vi "testCANopen.vi"() -> ()   [LabVIEW 2017, in "canopen.lvlib"]
doc: "Tests CANopen (and possibly CANbus) nets exercising the CANopen.lvclass APIs."
uses:
  canopen.lvlib
  CANopen/Multiplexor.ctl
  CANopen/FunctionCode.ctl
  DSP402/DSP402.lvclass
  CANopen/CANopen.lvclass
  DSP402/DriveState.ctl
  DSP402/DriveMode.ctl
  types/threestateFlag.ctl
panel:
  in  "CANopen":refnum<class "CANopen.lvclass">
  in  "DSP402":refnum<class "DSP402.lvclass">
  in  "Variant":variant=variant(u8[] [80, 0])
  in  "Tab Control":T1(tab)
  in  "NMT send":bool
  in  "Node ID (NMT)":u8=50 caption="Node ID"
  in  "Command specifier":u8(ring)=129 items=["Start remote node"=1, "Stop remote node"=2, "Enter pre-operational state"=128, "Reset node"=129, "Reset communication"=130]
  in  "SDO size":u8=2 caption="Bytes" format="%0d"
  in  "SDO read":bool
  in  "Multiplexor":T2={"Index"=4119, "Sub-index"=0} {"Sub-index" format="%02x"; "Index" format="%04x"}
  in  "SDO value":u32 caption="Value" format="%08x"
  in  "SDO write":bool
  in  "Node ID (SDO)":u8=50 caption="Node ID"
  in  "Remap TxPDO":bool
  in  "TxPDO map":cluster{"CobID":u32, "nBytes":u8}[](array[cluster])=[{"CobID"=434, "nBytes"=2}] {"CobID" format="%x"}
  out "Input image":bool[](array[boolean])
  in  "Remap RxPDO":bool
  in  "RxPDO map":cluster{"CobID":u32, "nBytes":u8}[](array[cluster])=[{"CobID"=562, "nBytes"=5}] {"CobID" format="%x"}
  in  "Output image":bool[](array[boolean])
  in  "Node ID (402)":u8 caption="Node ID"
  in  "State (402)":T3 caption="State"
  in  "Mode (402)":T4 caption="Mode" items=["Undefined"=0, "Profile Position Mode"=1, "Velocity Mode"=2, "Profile Velocity Mode"=3, "Torque Profile Mode"=4, "Homing Mode"=6, "Interpolated Position Mode"=7]
  in  "Position (402)":u32 caption="Position"
  in  "Speed (402)":i16=500 caption="Speed (RpM)"
  in  "Operation flags (402)":cluster{"ON":bool, "OFF":bool}[](array[cluster])=[{"ON"=FALSE, "OFF"=FALSE}, {"ON"=FALSE, "OFF"=FALSE}, {"ON"=FALSE, "OFF"=FALSE}, {"ON"=FALSE, "OFF"=FALSE}] caption="Force bit 4, 5, 6 and Halt"
  in  "Acceleration (402)":u32=100 caption="Acc"
  in  "Deceleration (402)":u32=100 caption="Dec"
  in  "Get status (402)":bool
  in  "PDO unlink":bool
  in  "PDO link":bool
  in  "Node ID (link)":u8=50 caption="Node ID"
  in  "Function code (link)":T5=4 caption="Function code" items=["NMT", "SYNC", "TIME STAMP", "EMERGENCY", "PDO1 (tx)", "PDO1 (rx)", "PDO2 (tx)", "PDO2 (rx)", "PDO3 (tx)", "PDO3 (rx)", "PDO4 (tx)", "PDO4 (rx)", "SDO (tx)", "SDO (rx)", "NMT Error Control"]
  in  "Indices":cluster{"Communication":u32, "Mapping":u32}={"Communication"=6144, "Mapping"=6656} {"Mapping" format="%x"; "Communication" format="%x"}
  in  "Map":cluster{"Multiplexor":T2, "nBits":u8}[](array[cluster])=[{"Multiplexor"={"Index"=24832, "Sub-index"=1}, "nBits"=16}] {"Multiplexor"."Sub-index" format="%02x"; "Multiplexor"."Index" format="%04x"}
  in  "Heartbeat set":bool
  in  "Heartbeat table":T6(array[cluster]) {"Period" format="%#.3g"}
  in  "Raw send":bool
  in  "Data (raw)":u8[](array[numeric]) caption="Data" format="%02x"
  in  "Node ID (raw)":u8 caption="Node ID"
  in  "Function code (raw)":T5=1 items=["NMT", "SYNC", "TIME STAMP", "EMERGENCY", "PDO1 (tx)", "PDO1 (rx)", "PDO2 (tx)", "PDO2 (rx)", "PDO3 (tx)", "PDO3 (rx)", "PDO4 (tx)", "PDO4 (rx)", "SDO (tx)", "SDO (rx)", "NMT Error Control"]
  in  "Stop":bool
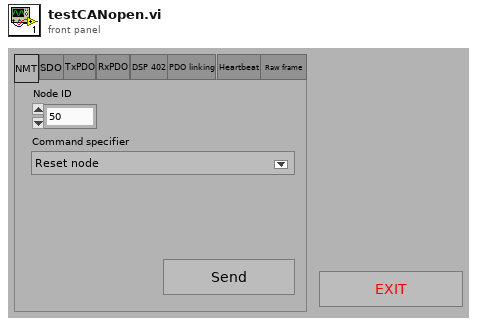
[diagram p1: front panel]
types:
  T1 = enum32{"NMT", "SDO", "TxPDO", "RxPDO", "DSP 402", "PDO linking", "Heartbeat", "Raw frame"}
  T2 = typedef "canopen.lvlib/CANopen.lvclass/Multiplexor.ctl" = cluster{"Index":u16, "Sub-index":u8}
  T3 = typedef "canopen.lvlib/DSP402.lvclass/DriveState.ctl" = enum16{"Start", "Not ready to switch on", "Switch on disabled", "Ready to switch on", "Switched on", "Operation enable", "Fault reaction active", "Fault", "Quick stop active"}
  T4 = typedef "canopen.lvlib/DSP402.lvclass/DriveMode.ctl" = i8
  T5 = typedef "canopen.lvlib/CANopen.lvclass/FunctionCode.ctl" = u8
  T6 = cluster{"Node ID":u8, "Period":dbl, "Set value":i16, "Value":i16}[]
  T7 = typedef "canopen.lvlib/threestateFlag.ctl" = i8
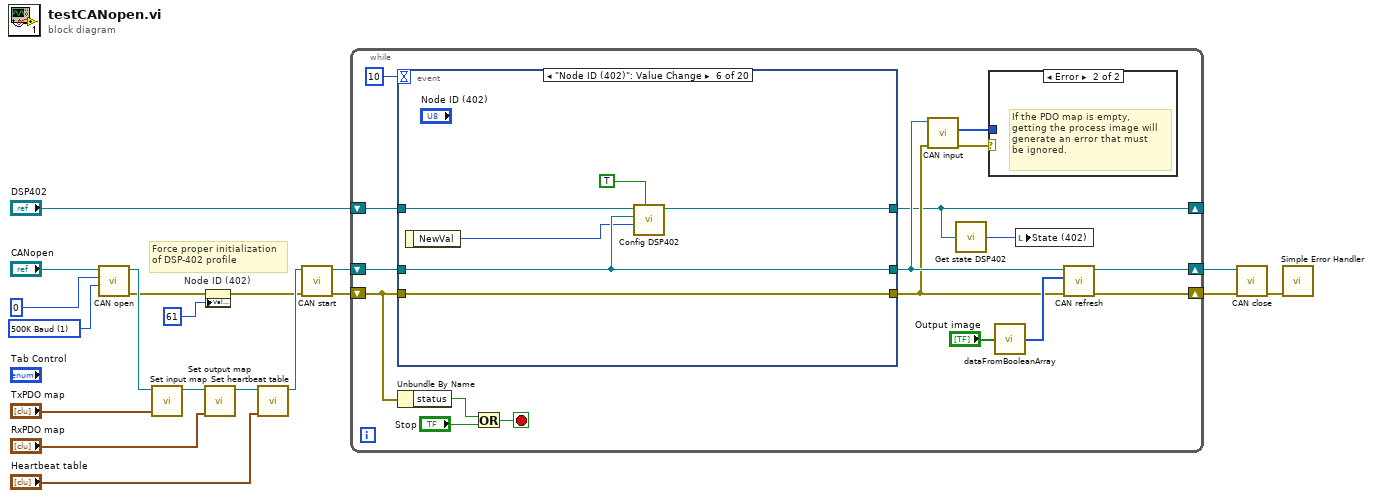
[diagram p0: block diagram]
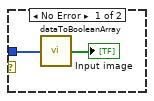
[diagram p2: hidden frame]
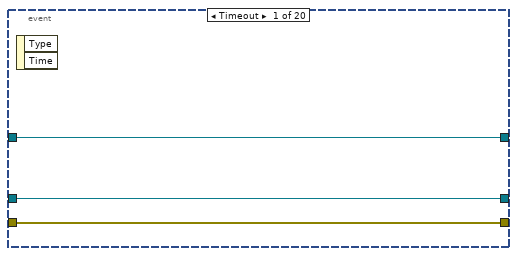
[diagram p3: hidden frame]
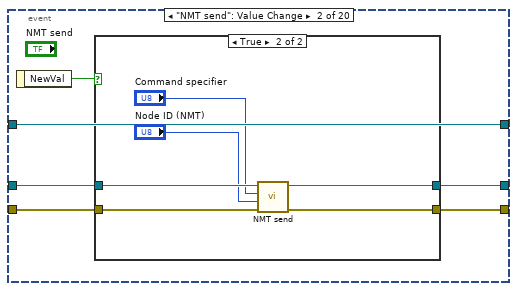
[diagram p4: hidden frame]
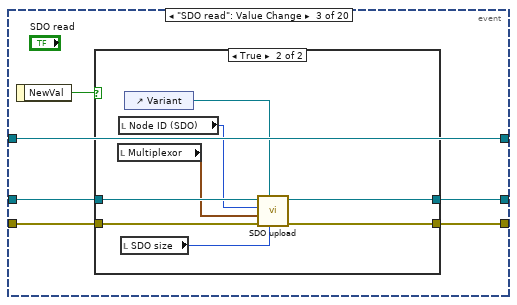
[diagram p6: hidden frame]
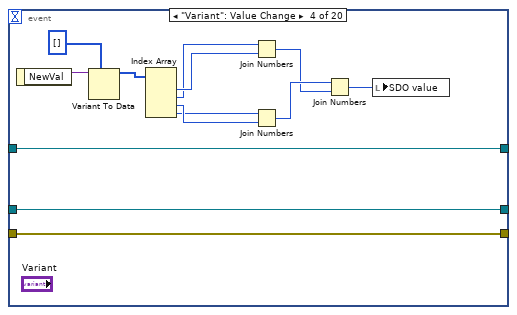
[diagram p8: hidden frame]
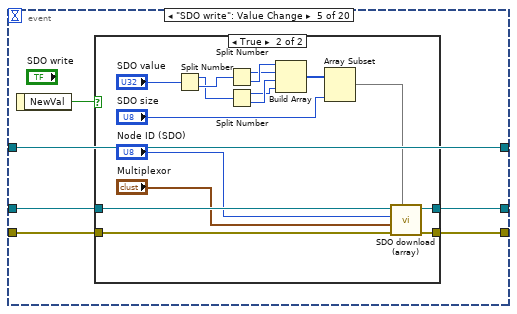
[diagram p9: hidden frame]
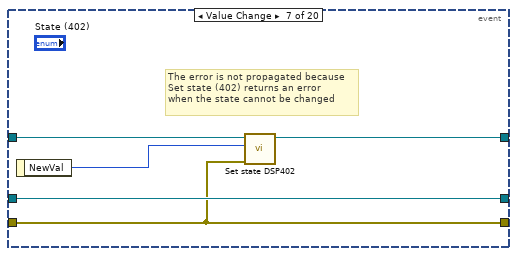
[diagram p11: hidden frame]
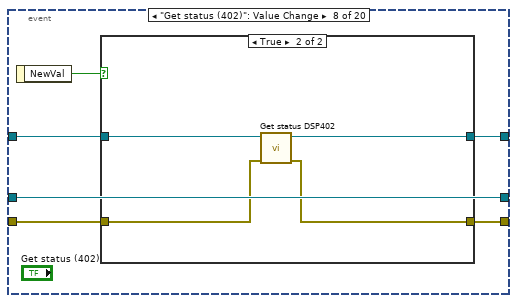
[diagram p12: hidden frame]
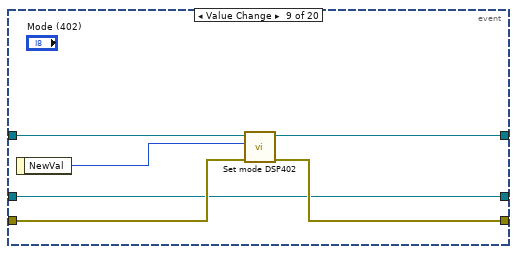
[diagram p14: hidden frame]
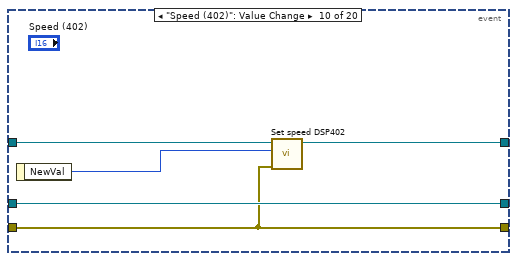
[diagram p15: hidden frame]
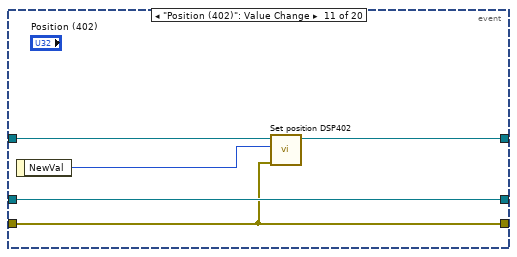
[diagram p16: hidden frame]
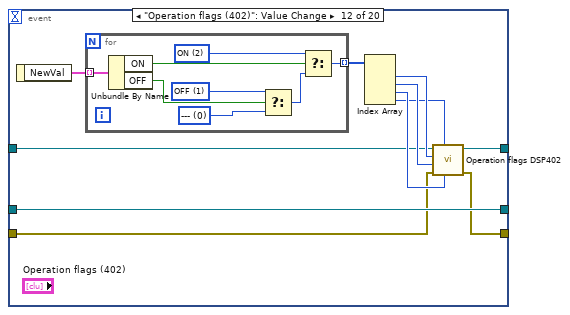
[diagram p17: hidden frame]
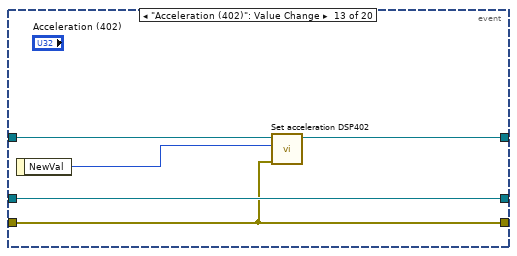
[diagram p18: hidden frame]
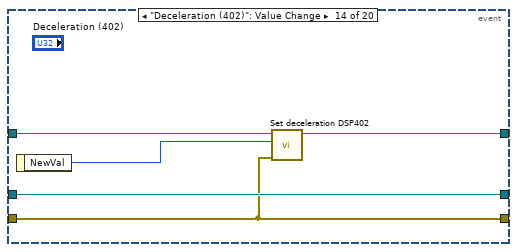
[diagram p19: hidden frame]
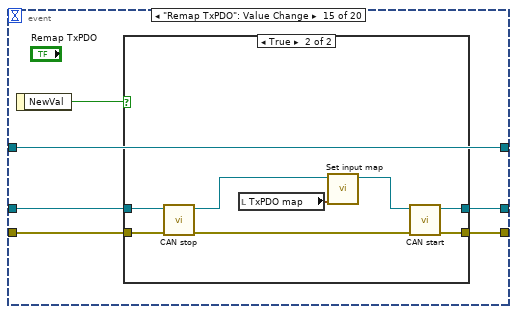
[diagram p20: hidden frame]
diagram:
  w15 = 1 items=["1M Baud", "500K Baud", "250K Baud", "125K Baud", "100K Baud", "62K Baud", "50K Baud"] ("Baud rate")
  # "Force proper initialization\nof DSP-402 profile"
  n1 = call "CAN open.vi"("Baud rate"=w15, "Channel"=u32 0, "CANopen in"="CANopen") -> ("error out"=w3:errorcluster, "CANopen out"=w11:refnum<class "CANopen.lvclass">)  [unwired: 1 in, 2 out]
  n2 = call "Set input map.vi"("Map"="TxPDO map", "CANopen in"=w11) -> ("CANopen out"=w10:refnum<class "CANopen.lvclass">)  [unwired: 5 out]
  n3 = call "Set output map.vi"("Map"="RxPDO map", "CANopen in"=w10) -> ("CANopen out"=w8:refnum<class "CANopen.lvclass">)  [unwired: 5 out]
  n4 = property on="Node ID (402)" class="DigNum (strict)"(error in=w3, "Val(Sgnl)"=u8 61 ("Value (Signaling)")) -> (error out=w2:errorcluster)  [unwired: 1 in, 1 out]
  n5 = call "Set heartbeat table.vi"("Heartbeat table"="Heartbeat table", "CANopen in"=w8) -> ("CANopen out"=w6:refnum<class "CANopen.lvclass">)  [unwired: 1 in, 4 out]
  n6 = call "CAN start.vi"("error in (no error)"=w2, "CANopen in"=w6) -> ("error out"=w5:errorcluster, "CANopen out"=w12:refnum<class "CANopen.lvclass">)  [unwired: 4 out]
  n7 = while {
    shift-right: [w26] -> w18
    shift-left: w5 -> [w34]
    shift-right: [w25] -> w19
    shift-left: w12 -> [w36]
    shift-right: [w21] -> _
    shift-left: "DSP402" -> [w22]
    stop <- w33 stop-if-true
    n8 = event shown="[5] \"Node ID (402)\": Value Change" {
      selector: _ -> [_ _ _ _ _ _ _ _ _ _ _ _ _ _ _ _ _ _ _ _]
      dyn-events: _ -> [_ _ _ _ _ _ _ _ _ _ _ _ _ _ _ _ _ _ _ _]
      timeout: 10 -> [_ _ _ _ _ _ _ _ _ _ _ _ _ _ _ _ _ _ _ _]
      tunnel: [w41 w47 w61 w84 w90 w112 w119 w120 w135 w142 w147 w157 w171 w176 w182 w198 w214 w226 w243 w259] -> w24
      tunnel: w36 -> [w41 w46 w60 w84 w89 w112 w119 w120 w135 w142 w147 w157 w171 w176 w181 w197 w213 w225 w242 w258]
      tunnel: [w40 w45 w59 w83 w88 w110 w115 w125 w136 w138 w143 w150 w167 w172 w180 w196 w212 w224 w241 w257] -> w23
      tunnel: w34 -> [w40 w44 w58 w83 w87 w110 w115 w124 w137 w138 w143 w151 w167 w172 w179 w195 w211 w223 w240 w256]
      tunnel: w22 -> [w39 w42 w56 w72 w85 w114 w117 w121 w133 w140 w146 w148 w169 w174 w177 w193 w209 w221 w238 w254]
      tunnel: [w39 w42 w56 w72 w85 w113 w116 w122 w132 w139 w145 w149 w168 w173 w177 w193 w209 w221 w238 w254] -> w21
      event Timeout {
        n9 = event-data() -> ()  [unwired: 3 out]
      }
      event "NMT send": Value Change {
        n10 = event-data() -> ("NewVal"=w43:bool)  [unwired: 1 out]
        n11 = case shown="True" w43 {
          tunnel: [w49 w52] -> w47
          tunnel: w46 -> [w49 w55]
          tunnel: [w48 w53] -> w45
          tunnel: w44 -> [w48 w54]
          frame False {
          }
          frame True {
            n12 = call "NMT send.vi"("error in (no error)"=w54, "Node ID"="Node ID (NMT)", "Command specifier"="Command specifier", "CANopen in"=w55) -> ("error out"=w53:errorcluster, "CANopen out"=w52:refnum<class "CANopen.lvclass">)  [unwired: 1 in, 1 out]
          }
        }
      }
      event "SDO read": Value Change {
        n13 = event-data() -> ("NewVal"=w57:bool)  [unwired: 1 out]
        n14 = case shown="True" w57 {
          tunnel: [w63 w68] -> w61
          tunnel: w60 -> [w63 w71]
          tunnel: [w62 w69] -> w59
          tunnel: w58 -> [w62 w70]
          frame False {
          }
          frame True {
            n15 = local read "Multiplexor"() -> (w66:T2)
            n16 = local read "Node ID (SDO)"() -> (w67:u8)
            n17 = local read "SDO size"() -> (w64:u8)
            n18 = control-ref of="Variant"() -> (w65:refnum<vi>)
            n19 = call "SDO upload.vi"("Size"=w64, "Destination"=w65, "error in (no error)"=w70, "Multiplexor"=w66, "Node ID"=w67, "CANopen in"=w71) -> ("error out"=w69:errorcluster, "CANopen out"=w68:refnum<class "CANopen.lvclass">)  [unwired: 2 out]
          }
        }
      }
      event "Variant": Value Change {
        n20 = event-data() -> ("NewVal"=w81:variant)  [unwired: 1 out]
        n21 = Variant To Data(type=u8[] [] ("Data"), Variant=w81) -> (data=w79:u8[])  [unwired: 1 in, 1 out]
        n22 = Index Array(array=w79) -> (element #1=w78:u8, element #2=w77:u8, element #3=w76:u8, element #4=w75:u8)  [unwired: 4 in]
        n23 = Join Numbers(hi=w77, lo=w78) -> ((hi.lo)=w73:u16)
        n24 = Join Numbers(hi=w75, lo=w76) -> ((hi.lo)=w74:u16)
        n25 = Join Numbers(hi=w74, lo=w73) -> ((hi.lo)=w80:u32)
        n26 = local write "SDO value"(w80) -> ()
      }
      event "SDO write": Value Change {
        n27 = event-data() -> ("NewVal"=w86:bool)  [unwired: 1 out]
        n28 = case shown="True" w86 {
          tunnel: [w92 w105] -> w90
          tunnel: w89 -> [w92 w108]
          tunnel: [w91 w106] -> w88
          tunnel: w87 -> [w91 w107]
          frame False {
          }
          frame True {
            n29 = Split Number(x="SDO value") -> (hi(x)=w99:u16, lo(x)=w101:u16)
            n30 = Split Number(x=w101) -> (hi(x)=w98:u8, lo(x)=w100:u8)
            n31 = Split Number(x=w99) -> (hi(x)=w96:u8, lo(x)=w97:u8)
            n32 = Build Array(w100, w98, w97, w96) -> (w95:u8[])
            n33 = Array Subset(array=w95, length="SDO size") -> (w93:u8[])  [unwired: 1 in]
            n34 = call "SDO download (array).vi"("Value"=w93, "error in (no error)"=w107, "Multiplexor"="Multiplexor", "Node ID"="Node ID (SDO)", "CANopen in"=w108) -> ("error out"=w106:errorcluster, "CANopen out"=w105:refnum<class "CANopen.lvclass">)  [unwired: 1 in, 2 out]
          }
        }
      }
      event "Node ID (402)": Value Change {
        n35 = event-data() -> ("NewVal"=w111:u8)  [unwired: 1 out]
        n36 = call "Config DSP402.vi"("Wait?"=TRUE, "Node ID"=w111, "CANopen"=w112, "DSP402 in"=w114) -> ("DSP402 out"=w113:refnum<class "DSP402.lvclass">)  [unwired: 1 in, 4 out]
      }
      event Value Change {
        # "The error is not propagated because\nSet state (402) returns an error\nwhen the state cannot be changed"
        n37 = event-data() -> ("NewVal"=w118:T3)  [unwired: 1 out]
        n38 = call "Set state DSP402.vi"("error in (no error)"=w115, "State"=w118, "DSP402 in"=w117) -> ("DSP402 out"=w116:refnum<class "DSP402.lvclass">)  [unwired: 4 out]
      }
      event "Get status (402)": Value Change {
        n39 = event-data() -> ("NewVal"=w123:bool)  [unwired: 1 out]
        n40 = case shown="True" w123 {
          tunnel: [w127 w130] -> w125
          tunnel: w124 -> [w127 w131]
          tunnel: [w126 w128] -> w122
          tunnel: w121 -> [w126 w129]
          frame False {
          }
          frame True {
            n41 = call "Get status DSP402.vi"("error in (no error)"=w131, "DSP402 in"=w129) -> ("error out"=w130:errorcluster, "DSP402 out"=w128:refnum<class "DSP402.lvclass">)  [unwired: 1 in, 3 out]
          }
        }
      }
      event Value Change {
        n42 = event-data() -> ("NewVal"=w134:T4)  [unwired: 1 out]
        n43 = call "Set mode DSP402.vi"("error in (no error)"=w137, "Mode"=w134, "DSP402 in"=w133) -> ("error out"=w136:errorcluster, "DSP402 out"=w132:refnum<class "DSP402.lvclass">)  [unwired: 3 out]
      }
      event "Speed (402)": Value Change {
        n44 = event-data() -> ("NewVal"=w141:i16)  [unwired: 1 out]
        n45 = call "Set speed DSP402.vi"("error in (no error)"=w138, "RpM"=w141, "DSP402 in"=w140) -> ("DSP402 out"=w139:refnum<class "DSP402.lvclass">)  [unwired: 8 out]
      }
      event "Position (402)": Value Change {
        n46 = event-data() -> ("NewVal"=w144:u32)  [unwired: 1 out]
        n47 = call "Set position DSP402.vi"("error in (no error)"=w143, "Position units"=w144, "DSP402 in"=w146) -> ("DSP402 out"=w145:refnum<class "DSP402.lvclass">)  [unwired: 3 in, 5 out]
      }
      event "Operation flags (402)": Value Change {
        n48 = event-data() -> ("NewVal"=w158:cluster{"ON":bool, "OFF":bool}[])  [unwired: 1 out]
        n49 = for {
          tunnel: w158 -> [w166] mode=indexing
          tunnel: [w160] -> w156 mode=indexing
          w164 = T7 2 items=["---", "OFF", "ON"] ("Flag")
          w161 = T7 1 items=["---", "OFF", "ON"] ("Flag")
          w159 = T7 0 items=["---", "OFF", "ON"] ("Flag")
          n50 = Unbundle By Name(w166) -> ("ON"=w165:bool, "OFF"=w163:bool)
          n51 = Select(t=w161, s=w163, f=w159) -> (s? t:f=w162:T7)
          n52 = Select(t=w164, s=w165, f=w162) -> (s? t:f=w160:T7)
        }
        n53 = Index Array(array=w156) -> (element #1=w155:T7, element #2=w154:T7, element #3=w153:T7, element #4=w152:T7)  [unwired: 4 in]
        n54 = call "Operation flags DSP402.vi"("Bit 6"=w153, "Halt"=w152, "error in (no error)"=w151, "Bit 5"=w154, "Bit 4"=w155, "DSP402 in"=w148) -> ("error out"=w150:errorcluster, "DSP402 out"=w149:refnum<class "DSP402.lvclass">)  [unwired: 4 out]
      }
      event "Acceleration (402)": Value Change {
        n55 = event-data() -> ("NewVal"=w170:u32)  [unwired: 1 out]
        n56 = call "Set acceleration DSP402.vi"("error in (no error)"=w167, "Acceleration units"=w170, "DSP402 in"=w169) -> ("DSP402 out"=w168:refnum<class "DSP402.lvclass">)  [unwired: 8 out]
      }
      event "Deceleration (402)": Value Change {
        n57 = event-data() -> ("NewVal"=w175:u32)  [unwired: 1 out]
        n58 = call "Set deceleration DSP402.vi"("error in (no error)"=w172, "Deceleration units"=w175, "DSP402 in"=w174) -> ("DSP402 out"=w173:refnum<class "DSP402.lvclass">)  [unwired: 8 out]
      }
      event "Remap TxPDO": Value Change {
        n59 = event-data() -> ("NewVal"=w178:bool)  [unwired: 1 out]
        n60 = case shown="True" w178 {
          tunnel: [w184 w191] -> w182
          tunnel: w181 -> [w184 w186]
          tunnel: [w183 w192] -> w180
          tunnel: w179 -> [w183 w189]
          frame False {
          }
          frame True {
            n61 = call "CAN stop.vi"("error in (no error)"=w189, "CANopen in"=w186) -> ("error out"=w188:errorcluster, "CANopen out"=w185:refnum<class "CANopen.lvclass">)  [unwired: 4 out]
            n62 = local read "TxPDO map"() -> (w187:cluster{"CobID":u32, "nBytes":u8}[])
            n63 = call "Set input map.vi"("Map"=w187, "CANopen in"=w185) -> ("CANopen out"=w190:refnum<class "CANopen.lvclass">)  [unwired: 5 out]
            n64 = call "CAN start.vi"("error in (no error)"=w188, "CANopen in"=w190) -> ("error out"=w192:errorcluster, "CANopen out"=w191:refnum<class "CANopen.lvclass">)  [unwired: 4 out]
          }
        }
      }
      event "Heartbeat set": Value Change {
        n65 = event-data() -> ("NewVal"=w194:bool)  [unwired: 1 out]
        n66 = case shown="True" w194 {
          tunnel: [w200 w207] -> w198
          tunnel: w197 -> [w200 w202]
          tunnel: [w199 w208] -> w196
          tunnel: w195 -> [w199 w205]
          frame False {
          }
          frame True {
            n67 = call "CAN stop.vi"("error in (no error)"=w205, "CANopen in"=w202) -> ("error out"=w204:errorcluster, "CANopen out"=w201:refnum<class "CANopen.lvclass">)  [unwired: 4 out]
            n68 = local read "Heartbeat table"() -> (w203:T6)
            n69 = call "Set heartbeat table.vi"("Heartbeat table"=w203, "CANopen in"=w201) -> ("CANopen out"=w206:refnum<class "CANopen.lvclass">)  [unwired: 5 out]
            n70 = call "CAN start.vi"("error in (no error)"=w204, "CANopen in"=w206) -> ("error out"=w208:errorcluster, "CANopen out"=w207:refnum<class "CANopen.lvclass">)  [unwired: 4 out]
          }
        }
      }
      event "Remap RxPDO": Value Change {
        n71 = event-data() -> ("NewVal"=w210:bool)  [unwired: 1 out]
        n72 = case shown="True" w210 {
          tunnel: [w216 w217] -> w214
          tunnel: w213 -> [w216 w219]
          tunnel: [w215 w218] -> w212
          tunnel: w211 -> [w215 w218]
          frame False {
          }
          frame True {
            n73 = local read "RxPDO map"() -> (w220:cluster{"CobID":u32, "nBytes":u8}[])
            n74 = call "Set output map.vi"("Map"=w220, "CANopen in"=w219) -> ("CANopen out"=w217:refnum<class "CANopen.lvclass">)  [unwired: 5 out]
          }
        }
      }
      event "PDO link": Value Change {
        n75 = event-data() -> ("NewVal"=w222:bool)  [unwired: 1 out]
        n76 = case shown="True" w222 {
          tunnel: [w228 w234] -> w226
          tunnel: w225 -> [w228 w237]
          tunnel: [w227 w235] -> w224
          tunnel: w223 -> [w227 w236]
          frame False {
          }
          frame True {
            n77 = call "enCOB-ID.vi"("Function code"="Function code (link)", "Node ID"="Node ID (link)") -> ("Cob ID"=w232:u32)
            n78 = call "PDO link.vi"("Map"="Map", "error in (no error)"=w236, "Indices"="Indices", "Cob ID"=w232, "CANopen in"=w237) -> ("error out"=w235:errorcluster, "CANopen out"=w234:refnum<class "CANopen.lvclass">)  [unwired: 1 in, 2 out]
          }
        }
      }
      event "PDO unlink": Value Change {
        n79 = event-data() -> ("NewVal"=w239:bool)  [unwired: 1 out]
        n80 = case shown="True" w239 {
          tunnel: [w245 w250] -> w243
          tunnel: w242 -> [w245 w253]
          tunnel: [w244 w251] -> w241
          tunnel: w240 -> [w244 w252]
          frame False {
          }
          frame True {
            n81 = local read "Function code (link)"() -> (w247:T5)
            n82 = local read "Node ID (link)"() -> (w248:u8)
            n83 = local read "Indices"() -> (w246:cluster{"Communication":u32, "Mapping":u32})
            n84 = call "enCOB-ID.vi"("Function code"=w247, "Node ID"=w248) -> ("Cob ID"=w249:u32)
            n85 = call "PDO unlink.vi"("error in (no error)"=w252, "Indices"=w246, "Cob ID"=w249, "CANopen in"=w253) -> ("error out"=w251:errorcluster, "CANopen out"=w250:refnum<class "CANopen.lvclass">)  [unwired: 1 in, 2 out]
          }
        }
      }
      event "Raw send": Value Change {
        n86 = event-data() -> ("NewVal"=w255:bool)  [unwired: 1 out]
        n87 = case shown="True" w255 {
          tunnel: [w261 w266] -> w259
          tunnel: w258 -> [w261 w269]
          tunnel: [w260 w267] -> w257
          tunnel: w256 -> [w260 w268]
          frame False {
          }
          frame True {
            n88 = call "enCOB-ID.vi"("Function code"="Function code (raw)", "Node ID"="Node ID (raw)") -> ("Cob ID"=w264:u32)
            n89 = call "CAN write.vi"("error in (no error)"=w268, "Data"="Data (raw)", "COB id"=w264, "CANopen in"=w269) -> ("error out"=w267:errorcluster, "CANopen out"=w266:refnum<class "CANopen.lvclass">)  [unwired: 1 in, 1 out]
          }
        }
      }
    }
    n90 = Unbundle By Name(w34) -> ("status"=w31:bool)
    n91 = Or(x=w31, y="Stop") -> (x .or. y?=w33:bool)
    n92 = call "CAN input.vi"("error in (no error)"=w23, "CANopen"=w24) -> ("error out"=w30:errorcluster, "Input image"=w29:u8[])  [unwired: 8 out]
    n93 = call-dynamic "Get state DSP402.vi"("DSP402 in"=w21) -> ("State"=w20:T3)
    n94 = case shown="Error" w30 {
      tunnel: w29 -> [w37 _]
      frame No Error {
        n95 = call "dataToBooleanArray.vi"("Data"=w37) -> ("Boolean array"=→"Input image":bool[])
      }
      frame Error {
        # "If the PDO map is empty,\ngetting the process image will\ngenerate an error that must\nbe ignored."
      }
    }
    n96 = call "dataFromBooleanArray.vi"("Boolean array"="Output image") -> ("Data"=w27:u8[])
    n97 = local write "State (402)"(w20) -> ()
    n98 = call "CAN refresh.vi"("error in (no error)"=w23, "Output image"=w27, "CANopen in"=w24) -> ("error out"=w26:errorcluster, "CANopen out"=w25:refnum<class "CANopen.lvclass">)  [unwired: 1 in, 2 out]
  }
  n99 = call "CAN close.vi"("error in (no error)"=w18, "CANopen in"=w19) -> ("error out"=w17:errorcluster)  [unwired: 5 out]
  n100 = call <vilib>:"Simple Error Handler.vi"("error in (no error)"=w17) -> ()  [unwired: 1 in, 8 out]
